vi "LinearSystemId_CreateDCMotorSystem.vi"(9 "G":dbl, 10 "jKgMetersSquared":dbl, 11 "DCMOTOR":T1 {"Jr_KgM2" format="%13.5p"; "L_H" format="%13.5p"; "Kt_NMPerAmp" format="%13.5p"; "KvINV_RadPerSecPerVolt" format="%13.5p"; "R_Ohms" format="%13.5p"; "FreeSpeed_RadPerSec" format="%13.5p"; "FreeCurrent_Amps" format="%13.5p"; "StallCurrent_Amps" format="%13.5p"; "StallTorque_NM" format="%13.5p"; "nominalVoltage_Volts" format="%13.5p"}) -> (0 "Error":bool, 3 "Linearsystem":T2)   [LabVIEW 2019, in "Trajectory_Library.lvlib"]
doc: "Create a state-space model of a DC motor system. The states of the system are [angular position, angular velocity], inputs are [voltage], and outputs are [angular position, angular velocity].\n\nCreate a state-space model of a DC motor system. The states of the system are \n [angular position, \n angular velocity] \n\ninputs are \n [voltage]\nand outputs are \n [angular position, \n angular velocity].\nInputs: \n - motor -- The motor (or gearbox) attached to the arm.\n - jKgMetersSquared -- The moment of inertia J of the motor and attached load. (Must be > 0)\n - G -- The reduction between motor and drum, as a ratio of output to input. (Must be > 0)\n\nOutputs:\n - LinearSystem -- A LinearSystem representing the given characterized constants.\n - Error -- A boolean indicating an error occured creating the system. A value of TRUE indicates an error."
uses:
  Trajectory_Library.lvlib
  LINEAR_SYSTEM.ctl
  <vilib>/Analysis/Matrix/Datatypes/RealMatrix.ctl
  DCMOTOR.CTL
  MatrixHelper_CoerceSize.vi
  <vilib>/Analysis/7linalg.llb/Create Special Matrix.vi
  <vilib>/Analysis/7linalg.llb/Create Special Real Matrix.vi
  <vilib>/Analysis/Matrix/NI_Matrix.lvlib
panel:
  # "<States,States>"
  # "<States,Inputs>"
  # "<Outputs,States>"
  # "<Outputs,Inputs>"
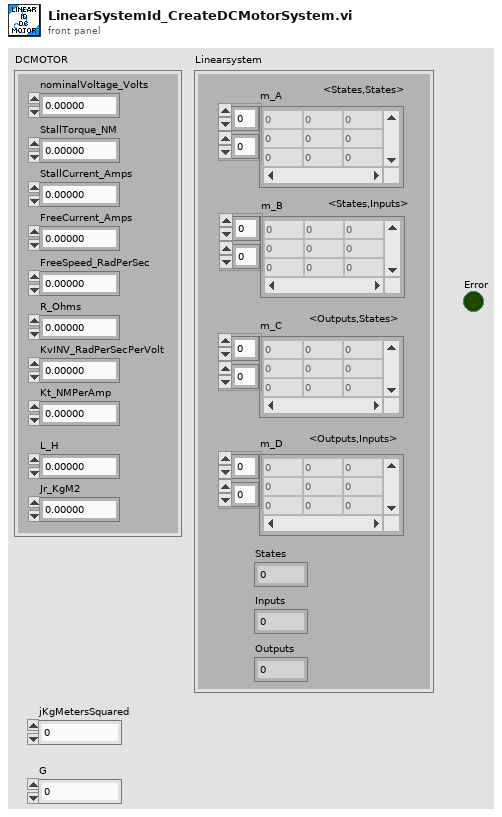
[diagram p1: front panel]
types:
  T1 = typedef "Trajectory_Library.lvlib/DCMOTOR.CTL" = cluster{"nominalVoltage_Volts":dbl, "StallTorque_NM":dbl, "StallCurrent_Amps":dbl, "FreeCurrent_Amps":dbl, "FreeSpeed_RadPerSec":dbl, "R_Ohms":dbl, "KvINV_RadPerSecPerVolt":dbl, "Kt_NMPerAmp":dbl, "L_H":dbl, "Jr_KgM2":dbl}
  T2 = typedef "Trajectory_Library.lvlib/LINEAR_SYSTEM.ctl" = cluster{"m_A":T3, "m_B":T3, "m_C":T3, "m_D":T3, "States":i32, "Inputs":i32, "Outputs":i32}
  T3 = typedef "NI_Matrix.lvlib/RealMatrix.ctl" = dbl[][]
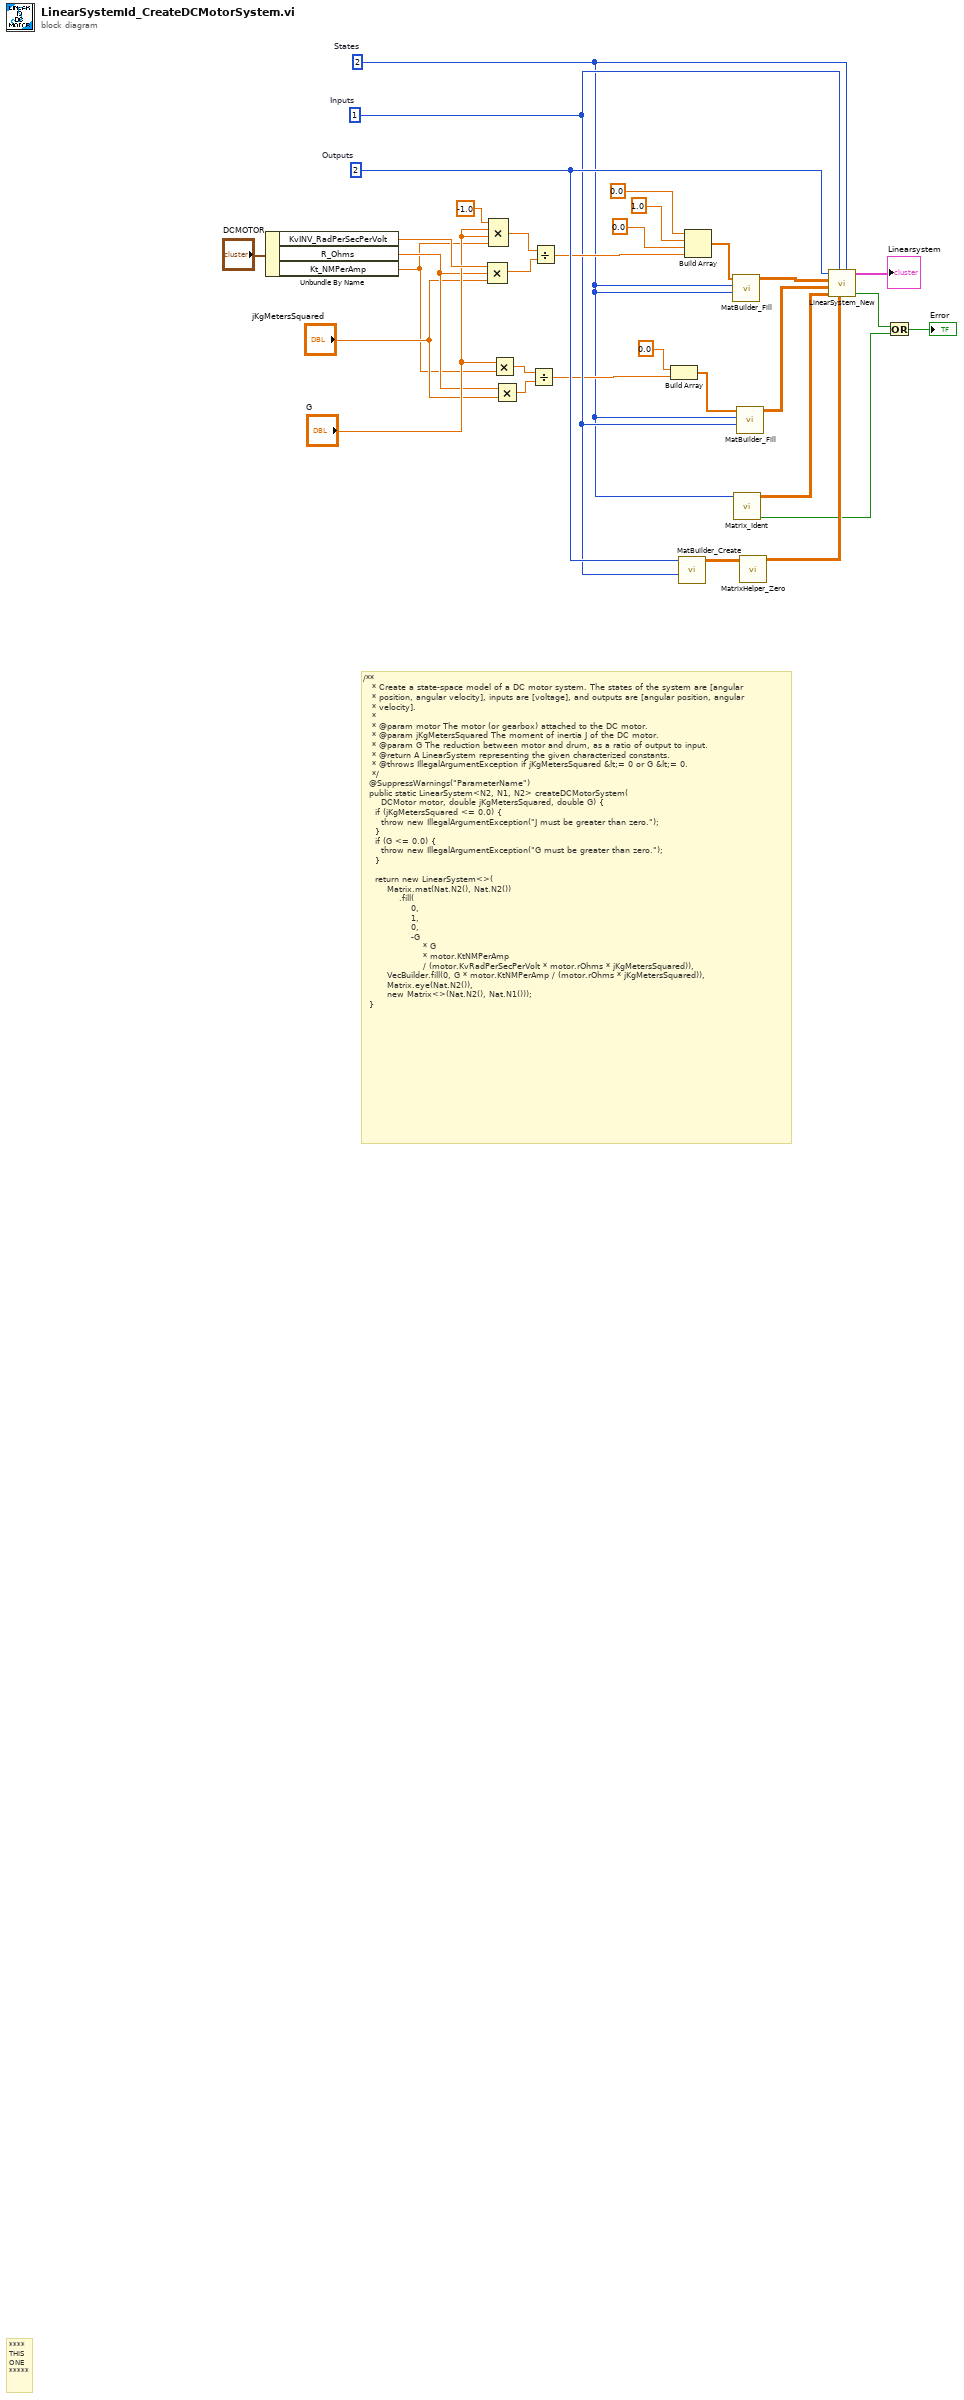
[diagram p0: block diagram]
diagram:
  w9 = 2  # States
  w12 = 1  # Inputs
  w19 = 2  # Outputs
  # "/**\n   * Create a state-space model of a DC motor system. The states of the system are [angular\n   * position, angular velocity], inputs are [voltage], and outputs are [angular position, angular\n   * velocity].\n   *\n   * @param motor The motor (or gearbox) attached to the DC motor.\n   * @param jKgMetersSquared The moment of inertia J of the DC motor.\n   * @param G The reduction between motor and drum, as a ratio of output to input.\n   * @return A LinearSystem representing the given characterized constants.\n   * @throws IllegalArgumentException if jKgMetersSquared &lt;= 0 or G &lt;= 0.\n   */\n  @SuppressWarnings(\"ParameterName\")\n  public static LinearSystem<N2, N1, N2> createDCMotorSystem(\n      DCMotor motor, double jKgMetersSquared, double G) {\n    if (jKgMetersSquared <= 0.0) {\n      throw new IllegalArgumentException(\"J must be greater than zero.\");\n    }\n    if (G <= 0.0) {\n      throw new IllegalArgumentException(\"G must be greater than zero.\");\n    }\n\n    return new LinearSystem<>(\n        Matrix.mat(Nat.N2(), Nat.N2())\n            .fill(\n                0,\n                1,\n                0,\n                -G\n                    * G\n                    * motor.KtNMPerAmp\n                    / (motor.KvRadPerSecPerVolt * motor.rOhms * jKgMetersSquared)),\n        VecBuilder.fill(0, G * motor.KtNMPerAmp / (motor.rOhms * jKgMetersSquared)),\n        Matrix.eye(Nat.N2()),\n        new Matrix<>(Nat.N2(), Nat.N1()));\n  }"
  # "****\nTHIS\nONE\n*****"
  n1 = Unbundle By Name("DCMOTOR") -> ("KvINV_RadPerSecPerVolt"=w28:dbl, "R_Ohms"=w24:dbl, "Kt_NMPerAmp"=w20:dbl)
  n2 = Compound Arithmetic op=MULTIPLY(w28, w24, "jKgMetersSquared") -> (w26:dbl)
  n3 = Compound Arithmetic op=MULTIPLY(-1.0 ("value"), "G", "G", w20) -> (w27:dbl)
  n4 = Multiply(x="G", y=w20) -> (x*y=w22:dbl)
  n5 = Multiply(x=w24, y="jKgMetersSquared") -> (x*y=w21:dbl)
  n6 = Divide(x=w22, y=w21) -> (x/y=w11:dbl)
  n7 = Divide(x=w27, y=w26) -> (x/y=w15:dbl)
  n8 = Build Array(0.0 ("element"), w11) -> (w13:dbl[])
  n9 = call "MatBuilder_Create.vi"("Columns"=w12, "Rows"=w19) -> ("output matrix"=w18:T3)  [unwired: 9 in]
  n10 = Build Array(0.0 ("element"), 1.0 ("element"), 0.0 ("element"), w15) -> (w16:dbl[])
  n11 = call "MatBuilder_Fill.vi"("Columns"=w9, "Rows"=w9, "Value List"=w16) -> ("output matrix"=w14:T3)  [unwired: 8 in]
  n12 = call "Matrix_Ident.vi"("Size"=w9) -> ("Error"=w7:bool, "output matrix"=w8:T3)  [unwired: 9 in]
  n13 = call "MatBuilder_Fill.vi"("Columns"=w12, "Rows"=w9, "Value List"=w13) -> ("output matrix"=w10:T3)  [unwired: 8 in]
  n14 = call "MatrixHelper_Zero.vi"("input matrix"=w18) -> ("output matrix"=w17:T3)  [unwired: 10 in]
  n15 = call "LinearSystem_New.vi"("States"=w9, "D"=w17, "Inputs"=w12, "C"=w8, "B"=w10, "A"=w14, "Outputs"=w19) -> ("Size Coerced"=w6:bool, "Linearsystem"=→"Linearsystem":T2)  [unwired: 3 in]
  n16 = Or(x=w6, y=w7) -> (x .or. y?=→"Error":bool)
